vi "Launch Config Module.vi"(8 "error in (no error)":errorcluster, 11 "Volatus Core in":refnum<class "Volatus Core.lvclass">) -> (0 "error out":errorcluster, 3 "Volatus Core out":refnum<class "Volatus Core.lvclass">)   [LabVIEW 2023, in "Volatus.lvlib" / "Volatus Core.lvclass"]
uses:
  Volatus Core.lvclass
  C:/dev/volatus/mts-volatus-super/libs/lv-volatus/Volatus/Module/Module.lvclass
  Config Type.ctl
  Volatus Core.lvclass/Volatus Core.ctl
  VolatusConfig/VolatusConfigElement/VolatusConfigElement.lvclass/VolatusConfigElement.ctl
  System Config Server/System Config Module.lvclass
  Module/Module.lvclass
  VolatusConfig/VolatusConfigElement/VolatusConfigElement.lvclass
  VolatusConfig/Node/Node Config.lvclass
  C:/dev/volatus/mts-volatus-super/libs/lv-volatus/VolatusConfig/VolatusConfigElement/VolatusConfigElement.lvclass
  C:/dev/volatus/mts-volatus-super/libs/lv-volatus/VolatusConfig/Node/Node Config.lvclass
  C:/dev/volatus/mts-volatus-super/libs/lv-volatus/Volatus/System Config Server/System Config Module.lvclass
  C:/dev/volatus/mts-volatus-super/libs/lv-volatus/Volatus/Volatus Core/Volatus Core.lvclass
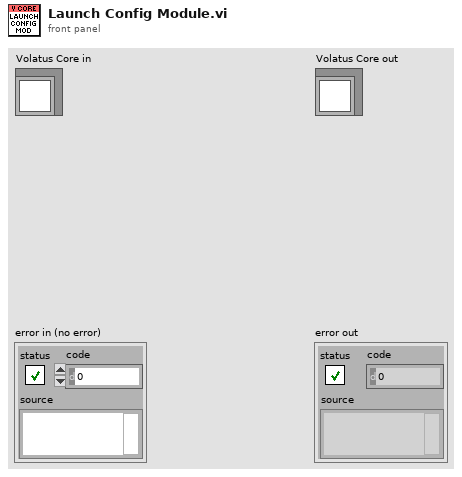
[diagram p1: front panel]
types:
  T1 = typedef "Volatus.lvlib/Volatus Core.lvclass/Config Type.ctl" = enum16{"App INI", "Memory", "Unconfigured"}
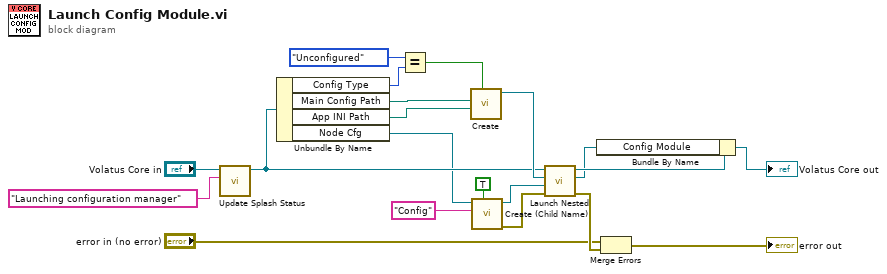
[diagram p0: block diagram]
diagram:
  n1 = call "Update Splash Status.vi"("Status"="Launching configuration manager", "Volatus Core in"="Volatus Core in") -> ("Volatus Core out"=w10:refnum<class "Volatus Core.lvclass">)  [unwired: 8 in, 1 out]
  n2 = Unbundle By Name(w10) -> ("Config Type"=w14:T1, "Main Config Path"=w16:path, "App INI Path"=w11:path, "Node Cfg"=w8:refnum<class "Node Config.lvclass">)
  n3 = Equal?(x=Config_Type."Unconfigured", y=w14) -> (x = y?=w12:bool)
  n4 = call "Create.vi"("Unconfigured"=w12, "INI Path"=w11, "Config Path"=w16) -> ("System Config Module out"=w15:refnum<class "System Config Module.lvclass">)  [unwired: 7 in, 1 out]
  n5 = call "Create (Child Name).vi"("Ignore Missing (F)"=TRUE, "Child Name"="Config", "Parent"=w8) -> ("error out"=w2:errorcluster, "VolatusConfigElement out"=w1:refnum<class "VolatusConfigElement.lvclass">)  [unwired: 7 in]
  n6 = call "Launch Nested.vi"("error in (no error)"=w2, "Config Element"=w1, "Nested Module"=w15, "Parent in"=w10) -> ("error out"=w6:errorcluster, "MessageQ"=w18:refnum<class "MessageQ.lvclass">, "Parent out"=w20:refnum<class "Volatus Core.lvclass">)  [unwired: 5 in]
  n7 = Bundle By Name(cluster=w20, "Config Module"=w18) -> (→"Volatus Core out":refnum<class "Volatus Core.lvclass">)
  n8 = Merge Errors("error in (no error)", w6) -> (→"error out":errorcluster)
